vi "波形记录处理V2.vi"(10 "控件配置文件":string[][](table), 11 "表格":string[][](table)) -> (1 "曲线数量":u16, 2 "曲线名称":string[](array[string]), 3 "波形图":dynamicdata(graph))   [LabVIEW 2021]
uses:
  controls/DataInitDef.ctl
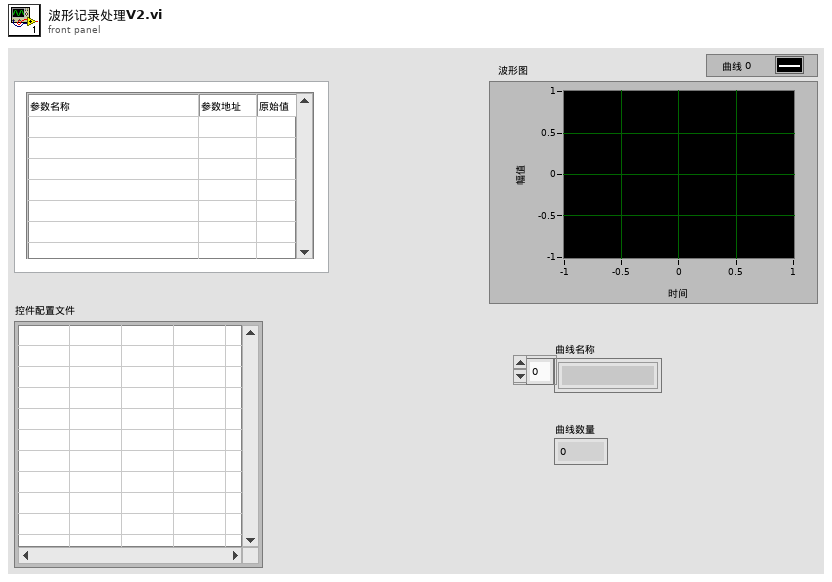
[diagram p1: front panel]
types:
  T1 = typedef "DataInitDef.ctl" = u16
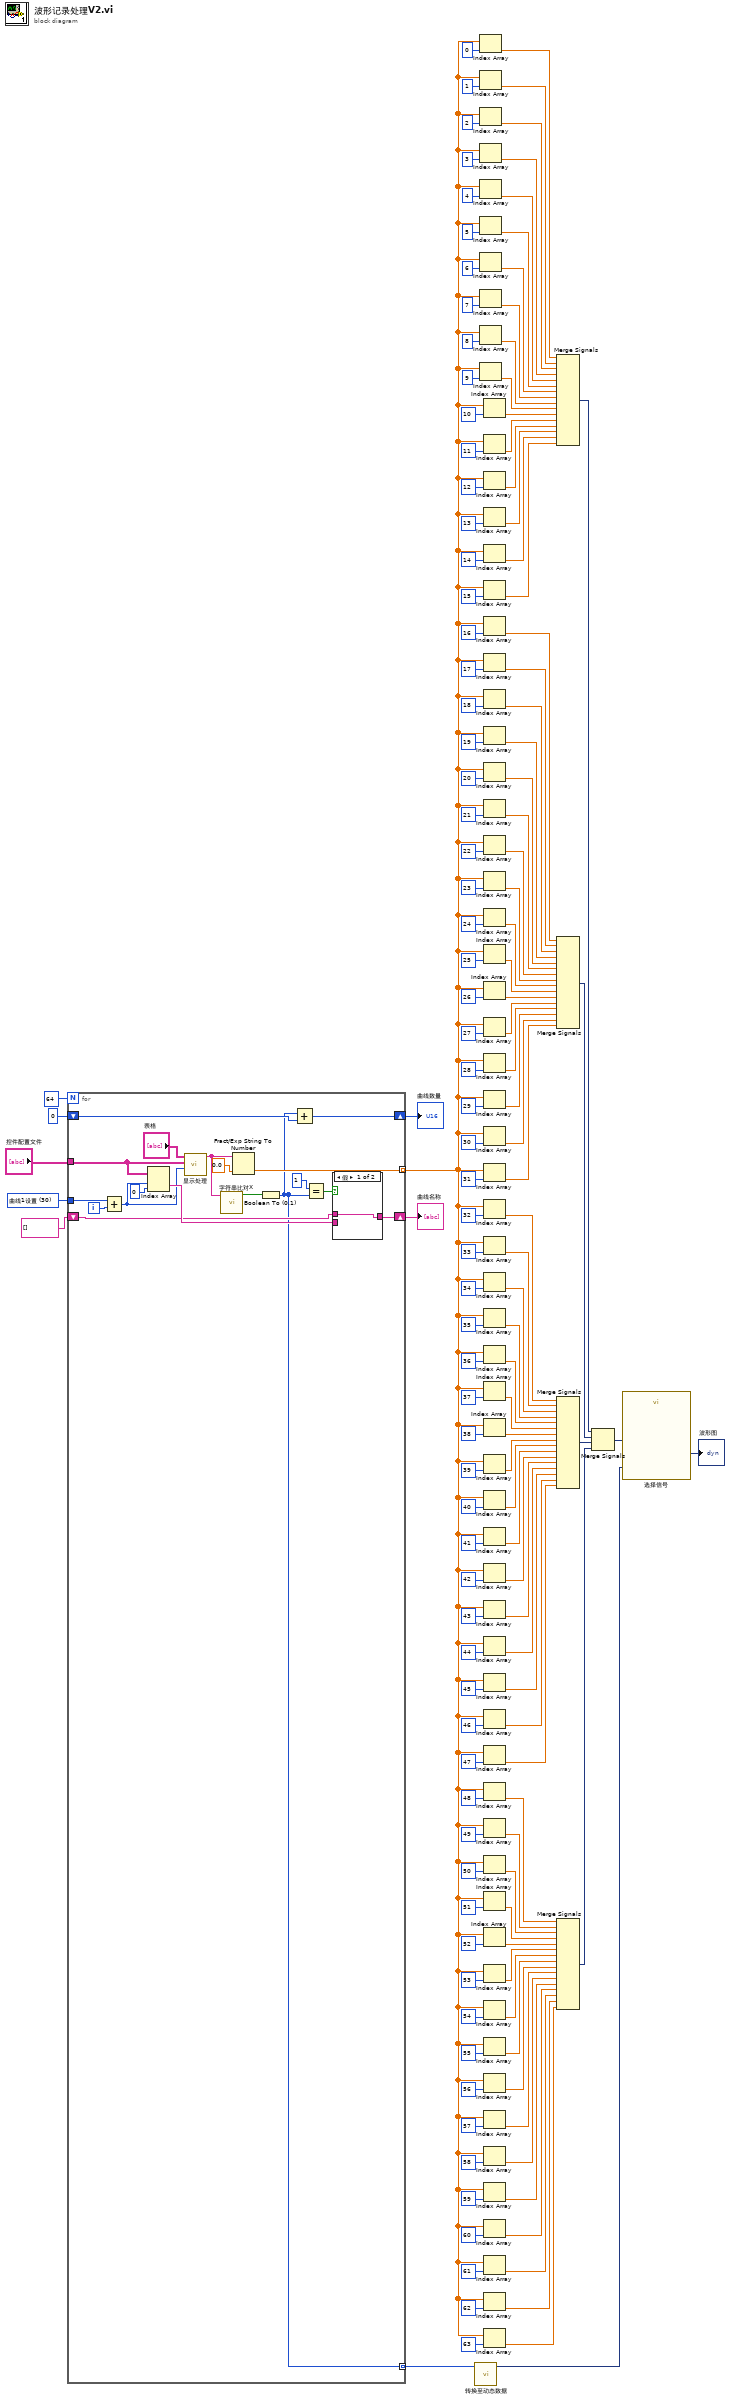
[diagram p0: block diagram]
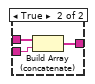
[diagram p2: hidden frame]
diagram:
  w143 = T1 30 items=["刷新间隔", "波特率", "布尔1设置项", "布尔2设置项", "布尔3设置项", "布尔4设置项", "布尔5设置项", "布尔6设置项", "布尔7设置项", "布尔8设置项", "显控1设置", "显控2设置", "显控3设置", "显控4设置", "显控5设置", "显控6设置", "显控7设置", "显控8设置", "显控9设置", "显控10设置", "显控11设置", "显控12设置", "设控1设置", "设控2设置", "设控3设置", "设控4设置", "设控5设置", "设控6设置", "设控7设置", "设控8设置", "曲线1设置", "曲线2设置", "曲线3设置", "曲线4设置", "曲线5设置", "曲线6设置", "曲线7设置", "曲线8设置", "曲线9设置", "曲线10设置", "曲线11设置", "曲线12设置", "曲线13设置", "曲线14设置", "曲线15设置", "曲线16设置", "曲线17设置", "曲线18设置", "曲线19设置", "曲线20设置", "曲线21设置", "曲线22设置", "曲线23设置", "曲线24设置", "曲线25设置", "曲线26设置", "曲线27设置", "曲线28设置", "曲线29设置", "曲线30设置", "曲线31设置", "曲线32设置", "曲线33设置", "曲线34设置", "曲线35设置", "曲线36设置", "曲线37设置", "曲线38设置", "曲线39设置", "曲线40设置", "曲线41设置", "曲线42设置", "曲线43设置", "曲线44设置", "曲线45设置", "曲线46设置", "曲线47设置", "曲线48设置", "曲线49设置", "曲线50设置", "曲线51设置", "曲线52设置", "曲线53设置", "曲线54设置", "曲线55设置", "曲线56设置", "曲线57设置", "曲线58设置", "曲线59设置", "曲线60设置", "曲线61设置", "曲线62设置", "曲线63设置", "曲线64设置", "ID值", "数据模式"] ("DataInitDef")
  n1 = for {
    N: 64 -> [_]
    tunnel: w143 -> [w148]
    tunnel: "控件配置文件" -> [w160]
    tunnel: [w145] -> w137 mode=indexing
    shift-right: [w156] -> w140
    shift-left: u16 0 -> [w155]
    shift-right: [w153] -> w138
    shift-left: string[] [] -> [w150]
    tunnel: [w146] -> w8 mode=indexing
    i -> [w149]
    n2 = Add(x=w148, y=w149) -> (x+y=w147:i32)
    n3 = Index Array(array=w160, index (row)=w147, index (col)=0 ("禁用的索引 (列)")) -> (element=w151:string)
    n4 = call "显示处理.vi"("项目"=w147, "配置文件"=w160, "表格"="表格") -> ("显示"=w158:string)  [unwired: 8 in]
    n5 = call "字符串比对X.vi"("字符串"=w158) -> ("布尔"=w157:bool)  [unwired: 10 in]
    n6 = Fract/Exp String To Number(string=w158, default (0 dbl)=0.0 ("默认(0 DBL)")) -> (number=w146:dbl)  [unwired: 2 in, 1 out]
    n7 = Boolean To (0,1)(Boolean=w157) -> (0, 1=w145:i16)
    n8 = Add(x=w145, y=w155) -> (x+y=w156:u16)
    n9 = Equal?(x=i16 1, y=w145) -> (x = y?=w152:bool)
    n10 = case shown="假" w152 {
      tunnel: [w163 w166] -> w153
      tunnel: w151 -> [_ w165]
      tunnel: w150 -> [w163 w164]
      frame False {
      }
      frame True {
        n11 = Build Array (concatenate)(w164, w165) -> (w166:string[])
      }
    }
  }
  "曲线数量" <- w140
  "曲线名称" <- w138
  n12 = call "转换至动态数据"("Array"=w137) -> ("Dynamic Data Type"=w136:dynamicdata)  [unwired: 3 in]
  n13 = Index Array(array=w8, index=0 ("索引")) -> (element=w133:dbl)
  n14 = Index Array(array=w8, index=1 ("索引")) -> (element=w130:dbl)
  n15 = Index Array(array=w8, index=2 ("索引")) -> (element=w129:dbl)
  n16 = Index Array(array=w8, index=3 ("索引")) -> (element=w68:dbl)
  n17 = Index Array(array=w8, index=4 ("索引")) -> (element=w62:dbl)
  n18 = Index Array(array=w8, index=5 ("索引")) -> (element=w67:dbl)
  n19 = Index Array(array=w8, index=6 ("索引")) -> (element=w66:dbl)
  n20 = Index Array(array=w8, index=7 ("索引")) -> (element=w65:dbl)
  n21 = Index Array(array=w8, index=8 ("索引")) -> (element=w64:dbl)
  n22 = Index Array(array=w8, index=9 ("索引")) -> (element=w63:dbl)
  n23 = Index Array(array=w8, index=10 ("索引")) -> (element=w61:dbl)
  n24 = Index Array(array=w8, index=11 ("索引")) -> (element=w60:dbl)
  n25 = Index Array(array=w8, index=12 ("索引")) -> (element=w59:dbl)
  n26 = Index Array(array=w8, index=13 ("索引")) -> (element=w58:dbl)
  n27 = Index Array(array=w8, index=14 ("索引")) -> (element=w57:dbl)
  n28 = Index Array(array=w8, index=15 ("索引")) -> (element=w56:dbl)
  n29 = Index Array(array=w8, index=16 ("索引")) -> (element=w55:dbl)
  n30 = Index Array(array=w8, index=17 ("索引")) -> (element=w54:dbl)
  n31 = Index Array(array=w8, index=18 ("索引")) -> (element=w53:dbl)
  n32 = Index Array(array=w8, index=19 ("索引")) -> (element=w52:dbl)
  n33 = Index Array(array=w8, index=20 ("索引")) -> (element=w51:dbl)
  n34 = Index Array(array=w8, index=21 ("索引")) -> (element=w50:dbl)
  n35 = Index Array(array=w8, index=22 ("索引")) -> (element=w49:dbl)
  n36 = Index Array(array=w8, index=23 ("索引")) -> (element=w48:dbl)
  n37 = Index Array(array=w8, index=24 ("索引")) -> (element=w47:dbl)
  n38 = Index Array(array=w8, index=25 ("索引")) -> (element=w46:dbl)
  n39 = Index Array(array=w8, index=26 ("索引")) -> (element=w45:dbl)
  n40 = Index Array(array=w8, index=27 ("索引")) -> (element=w44:dbl)
  n41 = Index Array(array=w8, index=28 ("索引")) -> (element=w43:dbl)
  n42 = Index Array(array=w8, index=29 ("索引")) -> (element=w42:dbl)
  n43 = Index Array(array=w8, index=30 ("索引")) -> (element=w41:dbl)
  n44 = Index Array(array=w8, index=31 ("索引")) -> (element=w40:dbl)
  n45 = Index Array(array=w8, index=32 ("索引")) -> (element=w39:dbl)
  n46 = Index Array(array=w8, index=33 ("索引")) -> (element=w38:dbl)
  n47 = Index Array(array=w8, index=34 ("索引")) -> (element=w37:dbl)
  n48 = Index Array(array=w8, index=35 ("索引")) -> (element=w36:dbl)
  n49 = Index Array(array=w8, index=36 ("索引")) -> (element=w35:dbl)
  n50 = Index Array(array=w8, index=37 ("索引")) -> (element=w34:dbl)
  n51 = Index Array(array=w8, index=38 ("索引")) -> (element=w33:dbl)
  n52 = Index Array(array=w8, index=39 ("索引")) -> (element=w32:dbl)
  n53 = Index Array(array=w8, index=40 ("索引")) -> (element=w31:dbl)
  n54 = Index Array(array=w8, index=41 ("索引")) -> (element=w30:dbl)
  n55 = Index Array(array=w8, index=42 ("索引")) -> (element=w29:dbl)
  n56 = Index Array(array=w8, index=43 ("索引")) -> (element=w28:dbl)
  n57 = Index Array(array=w8, index=44 ("索引")) -> (element=w27:dbl)
  n58 = Index Array(array=w8, index=45 ("索引")) -> (element=w26:dbl)
  n59 = Index Array(array=w8, index=46 ("索引")) -> (element=w25:dbl)
  n60 = Index Array(array=w8, index=47 ("索引")) -> (element=w24:dbl)
  n61 = Index Array(array=w8, index=48 ("索引")) -> (element=w23:dbl)
  n62 = Index Array(array=w8, index=49 ("索引")) -> (element=w22:dbl)
  n63 = Index Array(array=w8, index=50 ("索引")) -> (element=w21:dbl)
  n64 = Index Array(array=w8, index=51 ("索引")) -> (element=w20:dbl)
  n65 = Index Array(array=w8, index=52 ("索引")) -> (element=w19:dbl)
  n66 = Index Array(array=w8, index=53 ("索引")) -> (element=w18:dbl)
  n67 = Index Array(array=w8, index=54 ("索引")) -> (element=w17:dbl)
  n68 = Index Array(array=w8, index=55 ("索引")) -> (element=w16:dbl)
  n69 = Index Array(array=w8, index=56 ("索引")) -> (element=w15:dbl)
  n70 = Index Array(array=w8, index=57 ("索引")) -> (element=w14:dbl)
  n71 = Index Array(array=w8, index=58 ("索引")) -> (element=w13:dbl)
  n72 = Index Array(array=w8, index=59 ("索引")) -> (element=w12:dbl)
  n73 = Index Array(array=w8, index=60 ("索引")) -> (element=w11:dbl)
  n74 = Index Array(array=w8, index=61 ("索引")) -> (element=w10:dbl)
  n75 = Index Array(array=w8, index=62 ("索引")) -> (element=w7:dbl)
  n76 = Index Array(array=w8, index=63 ("索引")) -> (element=w6:dbl)
  n77 = Merge Signals(w133, w130, w129, w68, w62, w67, w66, w65, w64, w63, w61, w60, w59, w58, w57, w56) -> (w5:dynamicdata)
  n78 = Merge Signals(w55, w54, w53, w52, w51, w50, w49, w48, w47, w46, w45, w44, w43, w42, w41, w40) -> (w4:dynamicdata)
  n79 = Merge Signals(w39, w38, w37, w36, w35, w34, w33, w32, w31, w30, w29, w28, w27, w26, w25, w24) -> (w3:dynamicdata)
  n80 = Merge Signals(w23, w22, w21, w20, w19, w18, w17, w16, w15, w14, w13, w12, w11, w10, w7, w6) -> (w2:dynamicdata)
  n81 = Merge Signals(w5, w4, w3, w2) -> (w1:dynamicdata)
  n82 = call "选择信号"("Selector Input"=w136, "Signals"=w1) -> ("Signal Out"=→"波形图":dynamicdata)  [unwired: 8 in, 1 out]
